vi "Thor8000CheckEthernetResponse.vi"(1 "DataRead":string=":TEMP:ACT 9.51464272E+000\n", 2 "Data2Write":string=":slot 1;:temp:act? ") -> (0 "ReasonableResponse":bool)   [LabVIEW 2012]
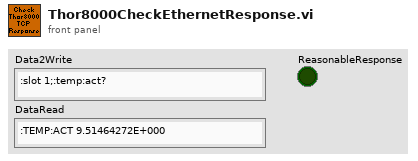
[diagram p1: front panel]
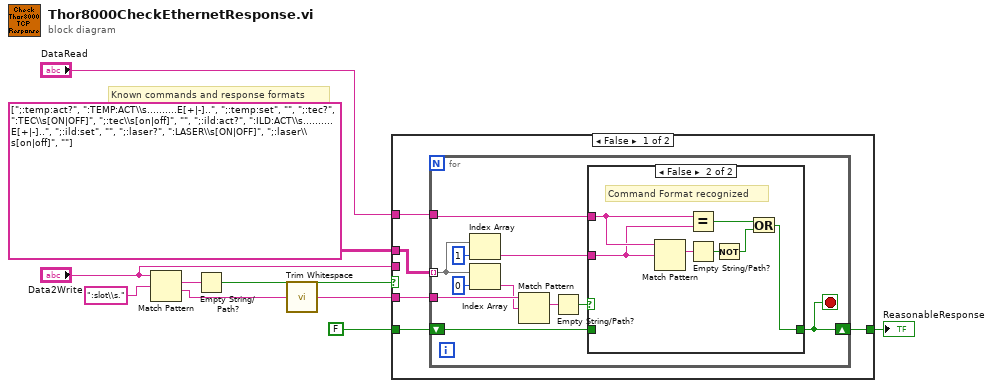
[diagram p0: block diagram]
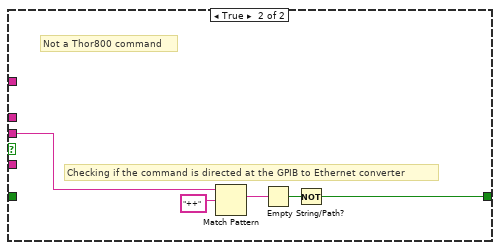
[diagram p3: hidden frame]
diagram:
  # "Known commands and response formats"
  n1 = Match Pattern(string="Data2Write", regular expression=":slot\\s.") -> (match substring=w9:string, after substring=w5:string)  [unwired: 1 in, 2 out]
  n2 = Empty String/Path?(string/path=w9) -> (empty?=w8:bool)
  n3 = call <vilib>:"Trim Whitespace.vi"("string"=w5) -> ("trimmed string"=w4:string)  [unwired: 1 in]
  n4 = case shown="False" w8 {
    tunnel: "DataRead" -> [w13 _]
    tunnel: w4 -> [w14 _]
    tunnel: string[][] [[";:temp:act?", ":TEMP:ACT\\s..........E[+|-].."], [";:temp:set", ""], [";:tec?", ":TEC\\s[ON|OFF]"], [";:tec\\s[on|off]", ""], [";:ild:act?", ":ILD:ACT\\s..........E[+|-].."], [";:ild:set", ""], [";:laser?", ":LASER\\s[ON|OFF]"], [";:laser\\s[on|off]", ""]] -> [w15 _]
    tunnel: FALSE -> [w12 _]
    tunnel: [w11 w35] -> w2
    tunnel: "Data2Write" -> [_ w39]
    frame False {
      n5 = for {
        tunnel: w15 -> [w23] mode=indexing
        tunnel: w14 -> [w18]
        tunnel: w13 -> [w21]
        shift-right: [w16] -> w11
        shift-left: w12 -> [w25]
        stop <- w16 stop-if-true
        n6 = Index Array(array=w23, index=1) -> (element=w22:string)
        n7 = Index Array(array=w23, index=0) -> (element=w17:string)
        n8 = Match Pattern(string=w18, regular expression=w17) -> (match substring=w20:string)  [unwired: 1 in, 3 out]
        n9 = Empty String/Path?(string/path=w20) -> (empty?=w19:bool)
        n10 = case shown="False" w19 {
          tunnel: w25 -> [w27 _]
          tunnel: [w27 w31] -> w16
          tunnel: w22 -> [_ w29]
          tunnel: w21 -> [_ w30]
          frame True {
            # "Command Format not recognized"
          }
          frame False {
            # "Command Format recognized"
            n11 = Match Pattern(string=w30, regular expression=w29) -> (match substring=w28:string)  [unwired: 1 in, 3 out]
            n12 = Equal?(x=w30, y=w29) -> (x = y?=w34:bool)
            n13 = Empty String/Path?(string/path=w28) -> (empty?=w33:bool)
            n14 = Not(x=w33) -> (.not. x?=w32:bool)
            n15 = Or(x=w34, y=w32) -> (x .or. y?=w31:bool)
          }
        }
      }
    }
    frame True {
      # "Checking if the command is directed at the GPIB to Ethernet converter"
      # "Not a Thor800 command"
      n16 = Match Pattern(string=w39, regular expression="++") -> (match substring=w37:string)  [unwired: 1 in, 3 out]
      n17 = Empty String/Path?(string/path=w37) -> (empty?=w36:bool)
      n18 = Not(x=w36) -> (.not. x?=w35:bool)
    }
  }
  "ReasonableResponse" <- w2
